vi "StringToCluster2(SubVI).vi"(10 "Проверка CRC8":bool, 11 "StringIn":string="xV4\u0012\u0002\u0000\u0000\u0000pМC\u0016њwѕa\u0000\u0000\u0001э\u0000\u0000\u0000\u0000\u0000\u0000\u0000\u0000\u0000\u0000\u0000\u0000\u0000\u0000\u0000\u0000\u0000\u0000\u0000\u0000o\u0012ѓ9\u0000\u0000\u0000\u0000\u0000\u0000\u0000\u0000+\u0019\u0000\u0000\u00002”И\u0000z\u0011") -> (2 "CRC8Good":bool, 3 "ECC_Cluster":T1={"MagicWord"=305419896, "FrameFormatVersion"=1, "Ncycle"=1, "Reserve"=3, "GlobalTime1"=4, "GlobalTime2"=5, "Reserve2"=6, "DataSize"=7, "CRC 8"=0, "EncodersParam1"=9, "EncodersParam2"=9, "LoseSamples"=10, "SamplingInterval"=1.0, "OverloadSamplesChannelX"=11, "OverloadSamplesChannelY"=12, "Reserve3"=13, "PacketCounter"=0, "Data1"=[[0.0, 0.0, 0.0, 0.0, 0.0, 0.0, 0.8999999999068677]]} {"PacketCounter" format="%08x"; "Reserve3" format="%08x"; "OverloadSamplesChannelY" format="%04x"; "OverloadSamplesChannelX" format="%04x"; "SamplingInterval" format="%#_6e"; "LoseSamples" format="%08x"; "EncodersParam2" format="%016x"; "EncodersParam1" format="%016x"; "CRC 8" format="%02x"; "Reserve2" format="%02x"; "Reserve" format="%02x"; "Ncycle" format="%04x"; "FrameFormatVersion" format="%02x"; "MagicWord" format="%.0x"})   [LabVIEW 2017]
uses:
  Control_EU/ClusterPack (Type).ctl
  <vilib>/Utility/error.llb/DialogType.ctl
panel:
  out "CRC8_CCITT":u8=171 format="%1x"
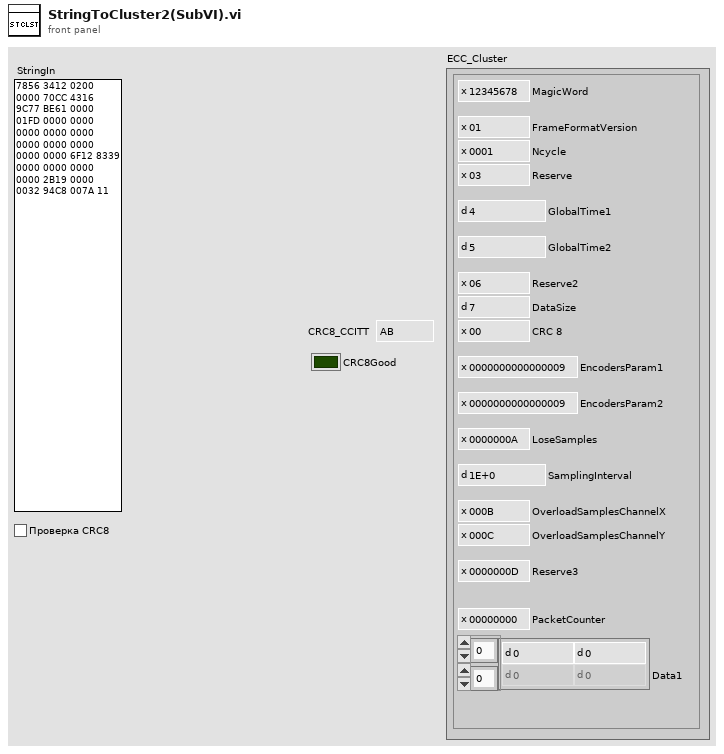
[diagram p1: front panel]
types:
  T1 = typedef "ClusterPack (Type).ctl" = cluster{"MagicWord":u32, "FrameFormatVersion":u8, "Ncycle":u16, "Reserve":u8, "GlobalTime1":u32, "GlobalTime2":u32, "Reserve2":u8, "DataSize":u16, "CRC 8":u8, "EncodersParam1":u64, "EncodersParam2":u64, "LoseSamples":u32, "SamplingInterval":sgl, "OverloadSamplesChannelX":u16, "OverloadSamplesChannelY":u16, "Reserve3":u32, "PacketCounter":u32, "Data1":dbl[][]}
  T2 = typedef "DialogType.ctl" = u16
  T3 = enum16{"big-endian, network order", "native, host order", "little-endian"}
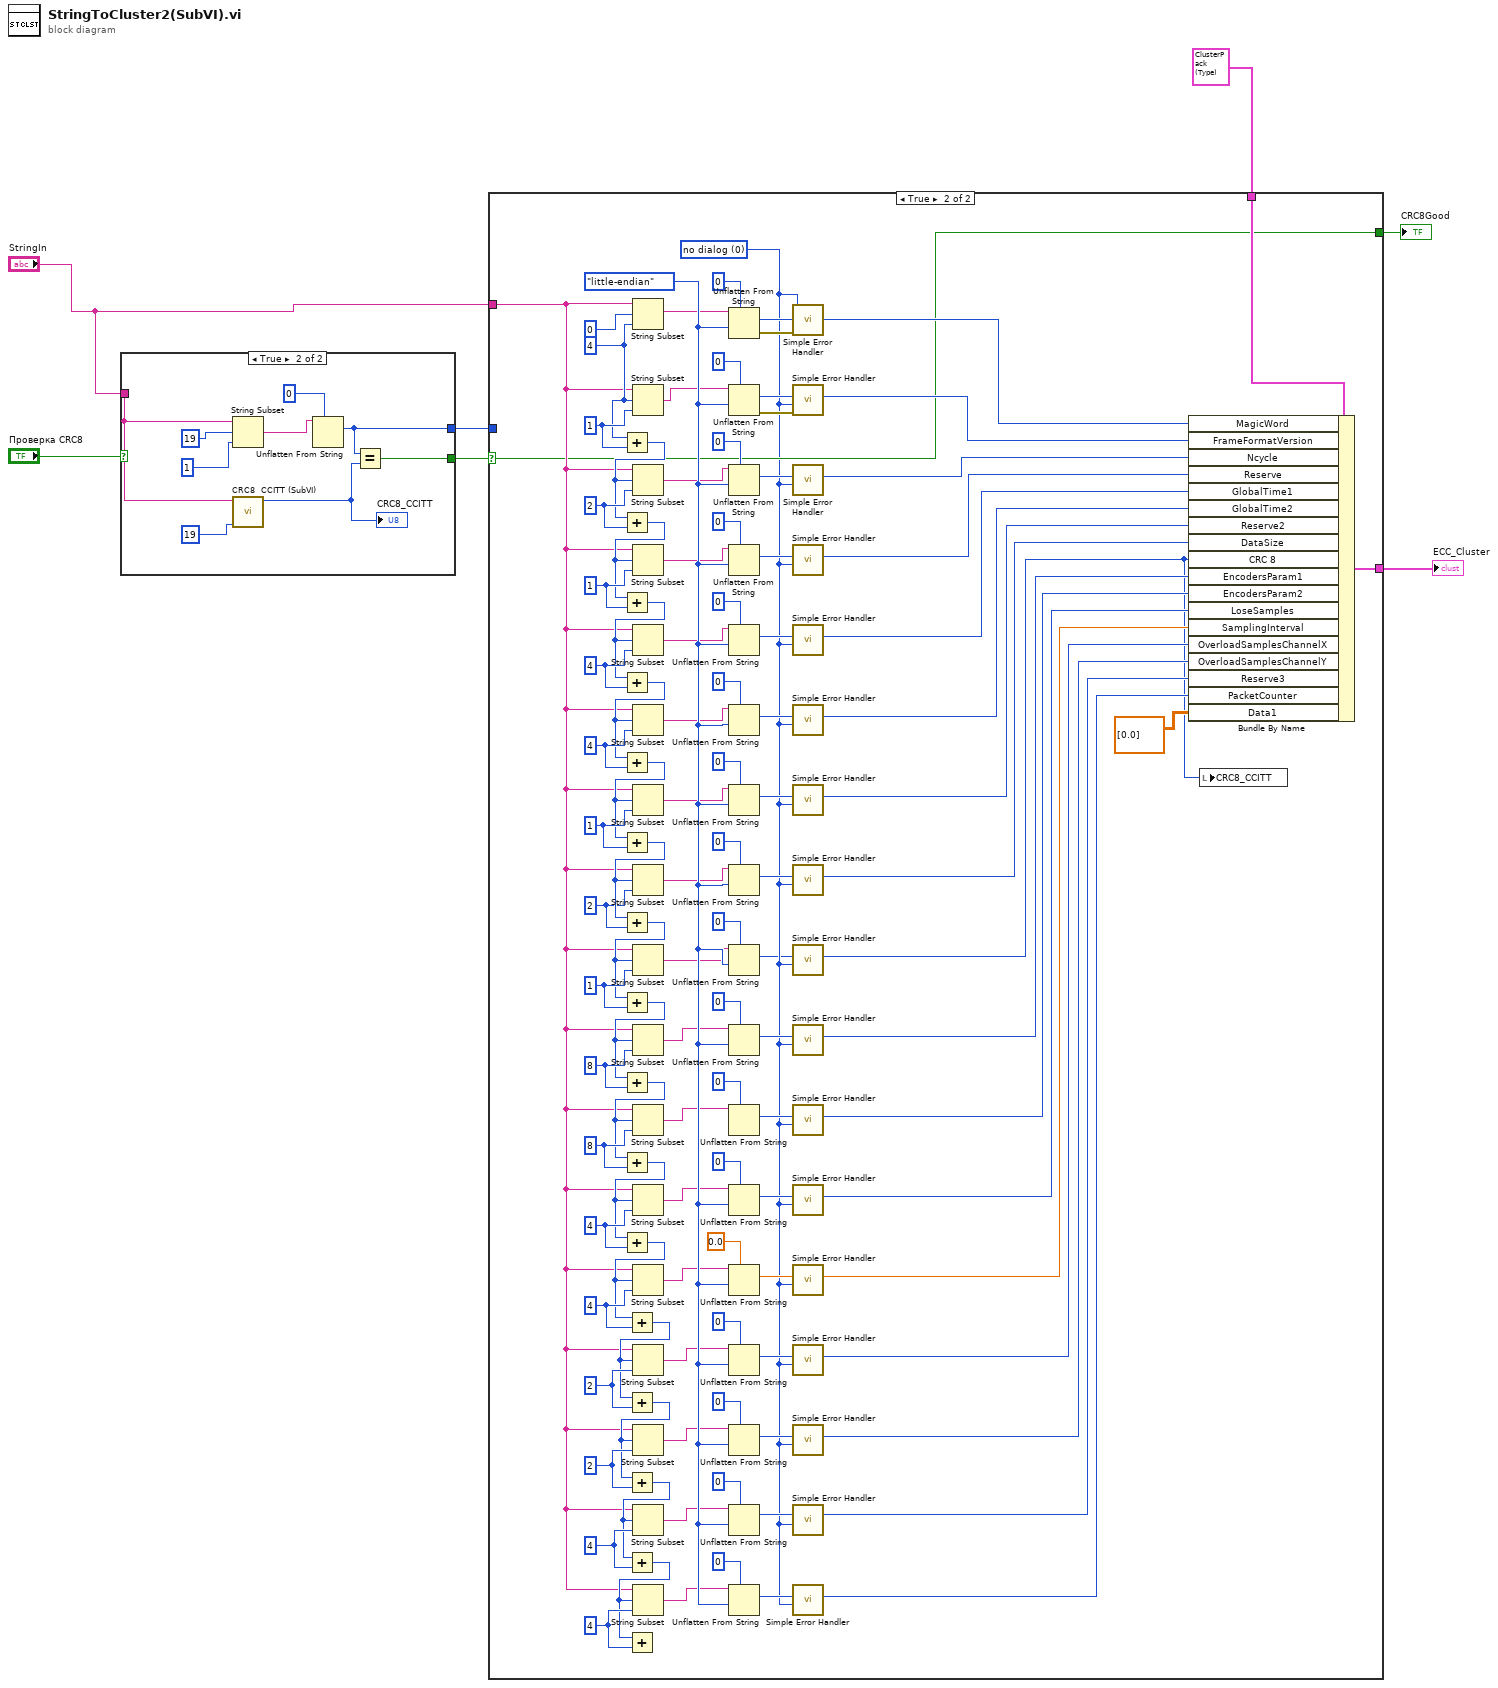
[diagram p0: block diagram]
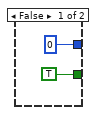
[diagram p2: hidden frame]
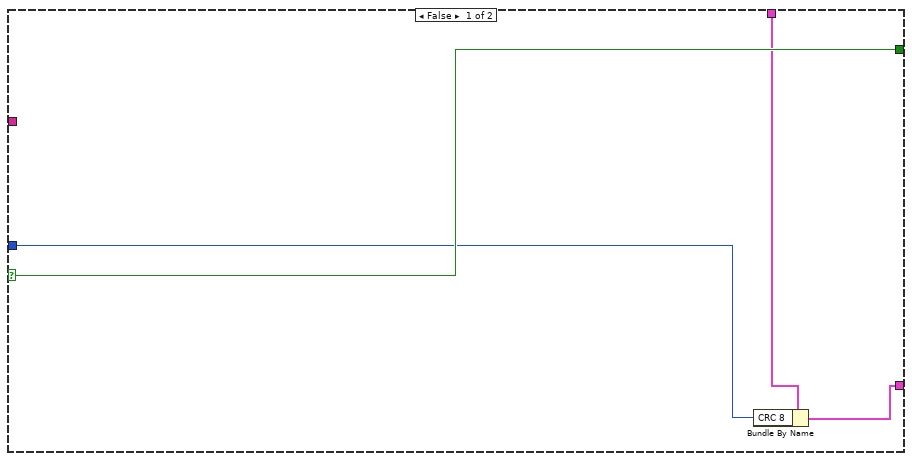
[diagram p3: hidden frame]
diagram:
  n1 = case shown="True" "Проверка CRC8" {
    tunnel: "StringIn" -> [_ w17]
    tunnel: [TRUE w11] -> w3
    tunnel: [u8 0 ("length (rest)") w10] -> w1
    frame False {
    }
    frame True {
      n2 = String Subset(string=w17, offset (0)=19, length (rest)=1 ("length (rest)")) -> (substring=w14:string)
      n3 = call "CRC8  CCITT (SubVI).vi"("wLength"=19 ("length (rest)"), "string in"=w17) -> ("CRC8_CCITT"=w12:u8)  [unwired: 9 in]
      "CRC8_CCITT" <- w12
      n4 = Unflatten From String(type=u8 0 ("length (rest)"), binary string=w14) -> (value=w10:u8)  [unwired: 3 in, 2 out]
      n5 = Equal?(x=w10, y=w12) -> (x = y?=w11:bool)
    }
  }
  n6 = case shown="True" w3 {
    selector: w3 -> [w22 w27]
    tunnel: T1 {"MagicWord"=0, "FrameFormatVersion"=0, "Ncycle"=0, "Reserve"=0, "GlobalTime1"=0, "GlobalTime2"=0, "Reserve2"=0, "DataSize"=0, "CRC 8"=0, "EncodersParam1"=0, "EncodersParam2"=0, "LoseSamples"=0, "SamplingInterval"=0.0, "OverloadSamplesChannelX"=0, "OverloadSamplesChannelY"=0, "Reserve3"=0, "PacketCounter"=0, "Data1"=[]} ("ECC_Cluster 5") -> [w21 w37]
    tunnel: [w20 w36] -> w7
    tunnel: "StringIn" -> [_ w28]
    tunnel: [w22 w27] -> w6
    tunnel: w1 -> [w19 _]
    frame False {
      n7 = Bundle By Name(cluster=w21, "CRC 8"=w19) -> (w20:T1)
    }
    frame True {
      w24 = T2 0 items=["no dialog", "OK message", "continue or stop message", "OK message + warnings", "continue/stop + warnings"] ("type of dialog (OK msg:1)")
      w113 = 4 ("length (rest)")
      w111 = 4 ("length (rest)")
      w105 = 2 ("length (rest)")
      w99 = 2 ("length (rest)")
      w97 = 4 ("length (rest)")
      w91 = 4 ("length (rest)")
      w83 = 8 ("length (rest)")
      w79 = 8 ("length (rest)")
      w72 = 1 ("length (rest)")
      w69 = 2 ("length (rest)")
      w66 = 1 ("length (rest)")
      w62 = 4 ("length (rest)")
      w114 = 4 ("length (rest)")
      w57 = 1 ("length (rest)")
      w49 = 2 ("length (rest)")
      w44 = 1 ("length (rest)")
      w108 = T3."little-endian" ("byte order (0:big-endian, network order)")
      w43 = 4 ("length (rest)")
      n8 = Add(x=w43, y=w44) -> (x+y=w48:i32)
      n9 = Add(x=w48, y=w49) -> (x+y=w52:i32)
      n10 = Add(x=w52, y=w57) -> (x+y=w56:i32)
      n11 = Add(x=w56, y=w114) -> (x+y=w61:i32)
      n12 = Add(x=w61, y=w62) -> (x+y=w65:i32)
      n13 = Add(x=w65, y=w66) -> (x+y=w70:i32)
      n14 = Add(x=w70, y=w69) -> (x+y=w71:i32)
      n15 = Add(x=w71, y=w72) -> (x+y=w78:i32)
      n16 = Add(x=w78, y=w79) -> (x+y=w82:i32)
      n17 = Add(x=w82, y=w83) -> (x+y=w86:i32)
      n18 = Add(x=w86, y=w91) -> (x+y=w90:i32)
      n19 = Add(x=w90, y=w97) -> (x+y=w98:i32)
      n20 = Add(x=w98, y=w99) -> (x+y=w104:i32)
      n21 = Add(x=w104, y=w105) -> (x+y=w110:i32)
      n22 = Add(x=w110, y=w111) -> (x+y=w112:i32)
      n23 = Add(x=w112, y=w113) -> ()  [unwired: 1 out]
      n24 = String Subset(string=w28, offset (0)=0, length (rest)=w43) -> (substring=w39:string)
      n25 = String Subset(string=w28, offset (0)=w43, length (rest)=w44) -> (substring=w42:string)
      n26 = String Subset(string=w28, offset (0)=w48, length (rest)=w49) -> (substring=w46:string)
      n27 = String Subset(string=w28, offset (0)=w52, length (rest)=w57) -> (substring=w47:string)
      n28 = String Subset(string=w28, offset (0)=w56, length (rest)=w114) -> (substring=w51:string)
      n29 = String Subset(string=w28, offset (0)=w61, length (rest)=w62) -> (substring=w55:string)
      n30 = String Subset(string=w28, offset (0)=w65, length (rest)=w66) -> (substring=w58:string)
      n31 = String Subset(string=w28, offset (0)=w70, length (rest)=w69) -> (substring=w64:string)
      n32 = String Subset(string=w28, offset (0)=w71, length (rest)=w72) -> (substring=w67:string)
      n33 = String Subset(string=w28, offset (0)=w78, length (rest)=w79) -> (substring=w74:string)
      n34 = String Subset(string=w28, offset (0)=w82, length (rest)=w83) -> (substring=w76:string)
      n35 = String Subset(string=w28, offset (0)=w86, length (rest)=w91) -> (substring=w88:string)
      n36 = String Subset(string=w28, offset (0)=w90, length (rest)=w97) -> (substring=w89:string)
      n37 = String Subset(string=w28, offset (0)=w98, length (rest)=w99) -> (substring=w93:string)
      n38 = String Subset(string=w28, offset (0)=w104, length (rest)=w105) -> (substring=w95:string)
      n39 = String Subset(string=w28, offset (0)=w110, length (rest)=w111) -> (substring=w101:string)
      n40 = String Subset(string=w28, offset (0)=w112, length (rest)=w113) -> (substring=w106:string)
      n41 = Unflatten From String(type=u32 0 ("MagicWord 2"), binary string=w39, byte order (0:big-endian, network order)=w108) -> (value=w34:u32, error out=w26:errorcluster)  [unwired: 2 in, 1 out]
      n42 = Unflatten From String(type=u8 0 ("MagicWord 2"), binary string=w42, byte order (0:big-endian, network order)=w108) -> (value=w33:u8, error out=w25:errorcluster)  [unwired: 2 in, 1 out]
      n43 = Unflatten From String(type=u16 0 ("MagicWord 2"), binary string=w46, byte order (0:big-endian, network order)=w108) -> (value=w32:u16)  [unwired: 2 in, 2 out]
      n44 = Unflatten From String(type=u8 0 ("MagicWord 2"), binary string=w47, byte order (0:big-endian, network order)=w108) -> (value=w31:u8)  [unwired: 2 in, 2 out]
      n45 = Unflatten From String(type=u32 0 ("MagicWord 2"), binary string=w51, byte order (0:big-endian, network order)=w108) -> (value=w30:u32)  [unwired: 2 in, 2 out]
      n46 = Unflatten From String(type=u32 0 ("MagicWord 2"), binary string=w55, byte order (0:big-endian, network order)=w108) -> (value=w29:u32)  [unwired: 2 in, 2 out]
      n47 = Unflatten From String(type=u8 0 ("MagicWord 2"), binary string=w58, byte order (0:big-endian, network order)=w108) -> (value=w60:u8)  [unwired: 2 in, 2 out]
      n48 = Unflatten From String(type=u16 0 ("MagicWord 2"), binary string=w64, byte order (0:big-endian, network order)=w108) -> (value=w115:u16)  [unwired: 2 in, 2 out]
      n49 = Unflatten From String(type=u8 0 ("MagicWord 2"), binary string=w67, byte order (0:big-endian, network order)=w108) -> (value=w23:u8)  [unwired: 2 in, 2 out]
      n50 = Unflatten From String(type=u64 0 ("MagicWord 2"), binary string=w74, byte order (0:big-endian, network order)=w108) -> (value=w75:u64)  [unwired: 2 in, 2 out]
      n51 = Unflatten From String(type=u64 0 ("MagicWord 2"), binary string=w76) -> (value=w80:u64)  [unwired: 3 in, 2 out]
      n52 = Unflatten From String(type=u32 0 ("MagicWord 2"), binary string=w88, byte order (0:big-endian, network order)=w108) -> (value=w84:u32)  [unwired: 2 in, 2 out]
      n53 = Unflatten From String(type=sgl 0.0 ("MagicWord 2"), binary string=w89, byte order (0:big-endian, network order)=w108) -> (value=w87:sgl)  [unwired: 2 in, 2 out]
      n54 = Unflatten From String(type=u16 0 ("MagicWord 2"), binary string=w93, byte order (0:big-endian, network order)=w108) -> (value=w94:u16)  [unwired: 2 in, 2 out]
      n55 = Unflatten From String(type=u16 0 ("MagicWord 2"), binary string=w95, byte order (0:big-endian, network order)=w108) -> (value=w102:u16)  [unwired: 2 in, 2 out]
      n56 = Unflatten From String(type=u32 0 ("MagicWord 2"), binary string=w101, byte order (0:big-endian, network order)=w108) -> (value=w103:u32)  [unwired: 2 in, 2 out]
      n57 = Unflatten From String(type=u32 0 ("MagicWord 2"), binary string=w106, byte order (0:big-endian, network order)=w108) -> (value=w109:u32)  [unwired: 2 in, 2 out]
      n58 = call <vilib>:"Simple Error Handler.vi"("type of dialog (OK msg:1)"=w24, "error in (no error)"=w26) -> ()  [unwired: 3 in, 5 out]
      n59 = call <vilib>:"Simple Error Handler.vi"("type of dialog (OK msg:1)"=w24, "error in (no error)"=w25) -> ()  [unwired: 3 in, 5 out]
      n60 = call <vilib>:"Simple Error Handler.vi"("type of dialog (OK msg:1)"=w24) -> ()  [unwired: 4 in, 5 out]
      n61 = call <vilib>:"Simple Error Handler.vi"("type of dialog (OK msg:1)"=w24) -> ()  [unwired: 4 in, 5 out]
      n62 = call <vilib>:"Simple Error Handler.vi"("type of dialog (OK msg:1)"=w24) -> ()  [unwired: 4 in, 5 out]
      n63 = call <vilib>:"Simple Error Handler.vi"("type of dialog (OK msg:1)"=w24) -> ()  [unwired: 4 in, 5 out]
      n64 = call <vilib>:"Simple Error Handler.vi"("type of dialog (OK msg:1)"=w24) -> ()  [unwired: 4 in, 5 out]
      n65 = call <vilib>:"Simple Error Handler.vi"("type of dialog (OK msg:1)"=w24) -> ()  [unwired: 4 in, 5 out]
      n66 = call <vilib>:"Simple Error Handler.vi"("type of dialog (OK msg:1)"=w24) -> ()  [unwired: 4 in, 5 out]
      n67 = call <vilib>:"Simple Error Handler.vi"("type of dialog (OK msg:1)"=w24) -> ()  [unwired: 4 in, 5 out]
      n68 = call <vilib>:"Simple Error Handler.vi"("type of dialog (OK msg:1)"=w24) -> ()  [unwired: 4 in, 5 out]
      n69 = call <vilib>:"Simple Error Handler.vi"("type of dialog (OK msg:1)"=w24) -> ()  [unwired: 4 in, 5 out]
      n70 = call <vilib>:"Simple Error Handler.vi"("type of dialog (OK msg:1)"=w24) -> ()  [unwired: 4 in, 5 out]
      n71 = call <vilib>:"Simple Error Handler.vi"("type of dialog (OK msg:1)"=w24) -> ()  [unwired: 4 in, 5 out]
      n72 = call <vilib>:"Simple Error Handler.vi"("type of dialog (OK msg:1)"=w24) -> ()  [unwired: 4 in, 5 out]
      n73 = call <vilib>:"Simple Error Handler.vi"("type of dialog (OK msg:1)"=w24) -> ()  [unwired: 4 in, 5 out]
      n74 = call <vilib>:"Simple Error Handler.vi"("type of dialog (OK msg:1)"=w24) -> ()  [unwired: 4 in, 5 out]
      n75 = Bundle By Name(cluster=w37, "MagicWord"=w34, "FrameFormatVersion"=w33, "Ncycle"=w32, "Reserve"=w31, "GlobalTime1"=w30, "GlobalTime2"=w29, "Reserve2"=w60, "DataSize"=w115, "CRC 8"=w23, "EncodersParam1"=w75, "EncodersParam2"=w80, "LoseSamples"=w84, "SamplingInterval"=w87, "OverloadSamplesChannelX"=w94, "OverloadSamplesChannelY"=w102, "Reserve3"=w103, "PacketCounter"=w109, "Data1"=dbl[][] [[0.0]]) -> (w36:T1)
      n76 = local write "CRC8_CCITT"(w23) -> ()
    }
  }
  "ECC_Cluster" <- w7
  "CRC8Good" <- w6
